vi "DAQ _ Create Data Queue.vi"(6 "如未找到则创建？(T)":bool=TRUE, 8 "error in":errorcluster caption="错误输入（无错误）", 11 "Q-name":string) -> (0 "error out":errorcluster, 3 "queue name":string)   [LabVIEW 2016]
uses:
  HardWare/Ctrls/HardWare _ Queue Data Type.ctl
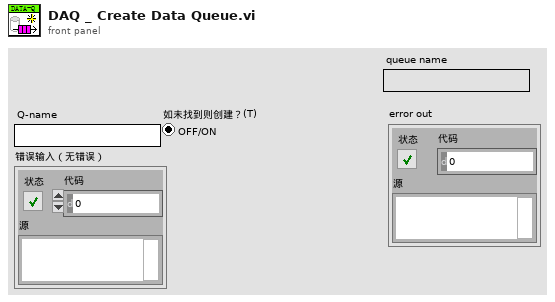
[diagram p1: front panel]
types:
  T1 = typedef "HardWare _ Queue Data Type.ctl" = cluster{"UnitNo.":i32, "data":dbl[][], "T0":dbl, "SampRate":dbl}
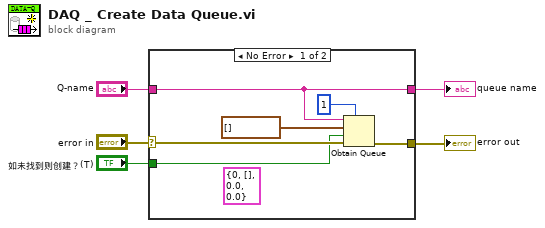
[diagram p0: block diagram]
diagram:
  n1 = case shown="No Error" "error in" {
    selector: "error in" -> [w11 w12]
    tunnel: "Q-name" -> [w8 _]
    tunnel: [w9 w12] -> w3
    tunnel: [w8 _] -> w2
    tunnel: "如未找到则创建？(T)" -> [w7 _]
    frame No Error {
      (unwired) T1 {"UnitNo."=0, "data"=[], "T0"=0.0, "SampRate"=0.0}
      n2 = Obtain Queue(max queue size (-1, unlimited)=1 ("队列最大值（-1，无限）"), name (unnamed)=w8, element data type=waveform(dbl)[] [] ("data"), create if not found? (T)=w7, error in (no error)=w11) -> (error out=w9:errorcluster)  [unwired: 2 out]
    }
    frame Error {
    }
  }
  "error out" <- w3
  "queue name" <- w2
